vi "finishUI.vi"(8 "error in (no error)":errorcluster, 11 "UI in":refnum<class "UI.lvclass">) -> (0 "error out":errorcluster)   [LabVIEW 2018, in "UI.lvclass"]
doc: "This VI closes the UI references and communicaton with Emedded VIs."
uses:
  UI.lvclass
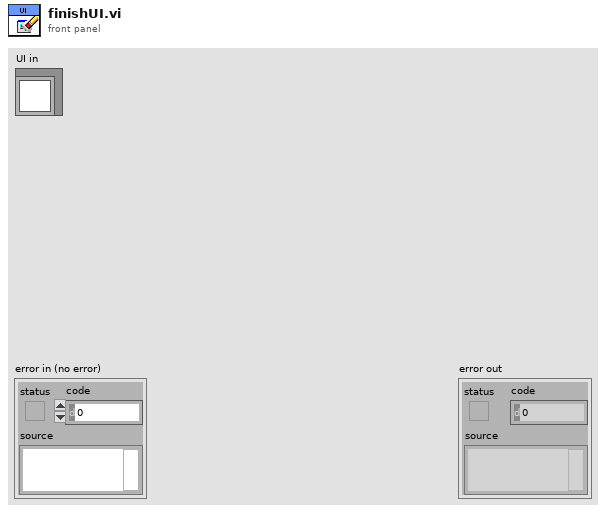
[diagram p1: front panel]
types:
  T1 = enum16{"Create", "Register", "Generate", "Unregister", "Destroy"}
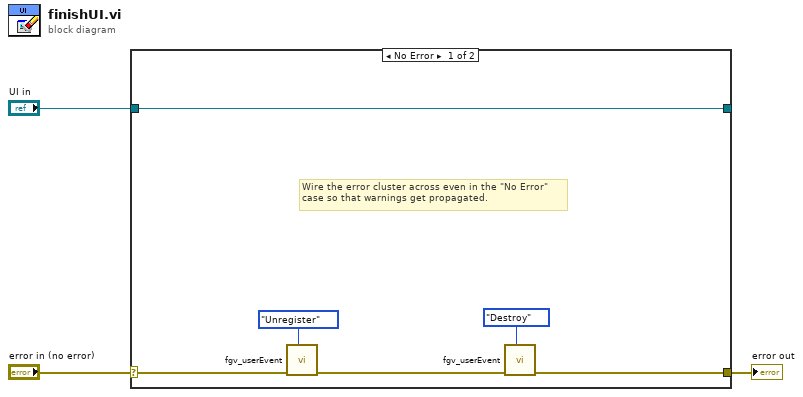
[diagram p0: block diagram]
diagram:
  n1 = case shown="No Error" "error in (no error)" {
    selector: "error in (no error)" -> [w8 w11]
    tunnel: [w6 w11] -> w2
    tunnel: [w9 w10] -> _
    tunnel: "UI in" -> [w9 w10]
    frame No Error {
      # "Wire the error cluster across even in the \"No Error\"\ncase so that warnings get propagated."
      n2 = call "fgv_userEvent.vi"("Option"=T1."Unregister", "Error In"=w8) -> ("Error Out"=w7:errorcluster)  [unwired: 8 in, 1 out]
      n3 = call "fgv_userEvent.vi"("Option"=T1."Destroy", "Error In"=w7) -> ("Error Out"=w6:errorcluster)  [unwired: 8 in, 1 out]
    }
    frame Error {
    }
  }
  "error out" <- w2
